vi "Set Document Reference.vi"(8 "error in (no error)":errorcluster, 9 "Document":refnum<k24>, 11 "ooDocument in":refnum<class "ooDocument.lvclass">) -> (0 "error out":errorcluster, 3 "ooDocument out":refnum<class "ooDocument.lvclass">)   [LabVIEW 2009, in "ooDocument.lvclass"]
uses:
  ooDocument.lvclass
  C:/Projets/LAVAG/OpenOfficeRGT/AODL/DLLs/AODL.dll
  ooDocument.lvclass/ooDocument.ctl
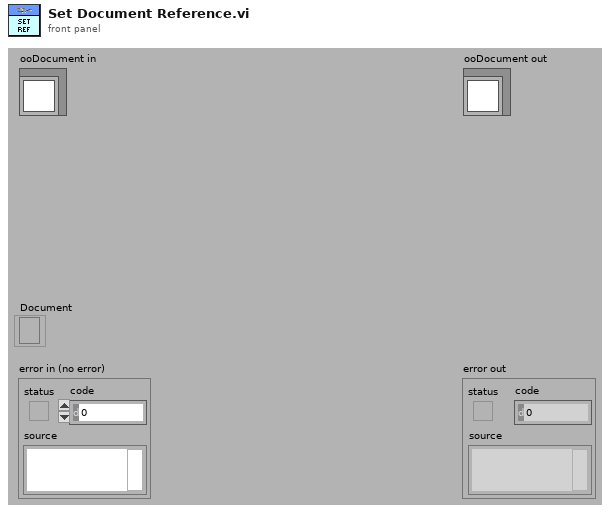
[diagram p1: front panel]
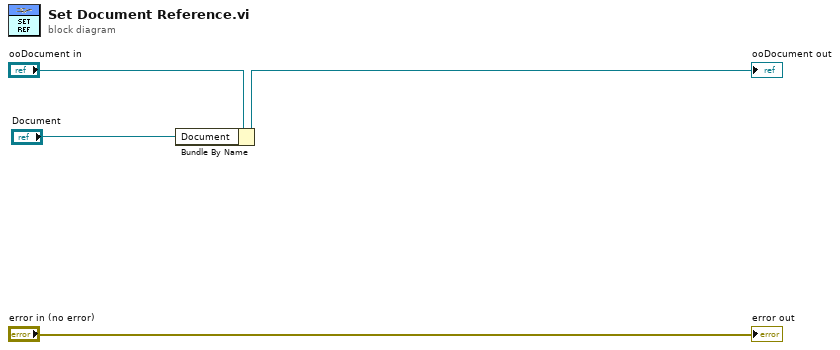
[diagram p0: block diagram]
diagram:
  n1 = Bundle By Name(cluster="ooDocument in", "Document"="Document") -> (→"ooDocument out":refnum<class "ooDocument.lvclass">)
  "error out" <- "error in (no error)"
